vi "SwitchOption.vi"(6 "SubPanelRef":refnum<vi>, 7 "Panel Controller":refnum<class "MemberPanel.lvclass">, 8 "error in (no error)":errorcluster, 9 "Base Path":path, 10 "ThreadName(\"\")":string, 11 "Admin_Actor in":refnum<class "Admin_Actor.lvclass">) -> (0 "error out":errorcluster, 3 "Admin_Actor out":refnum<class "Admin_Actor.lvclass">)   [LabVIEW 2015, in "Admin_Actor.lvlib" / "Admin_Actor.lvclass"]
uses:
  Admin_Actor.lvclass
  Member_Actor/MemberPanel/MemberPanel.lvclass
  Admin_Actor.lvclass/Admin_Actor.ctl
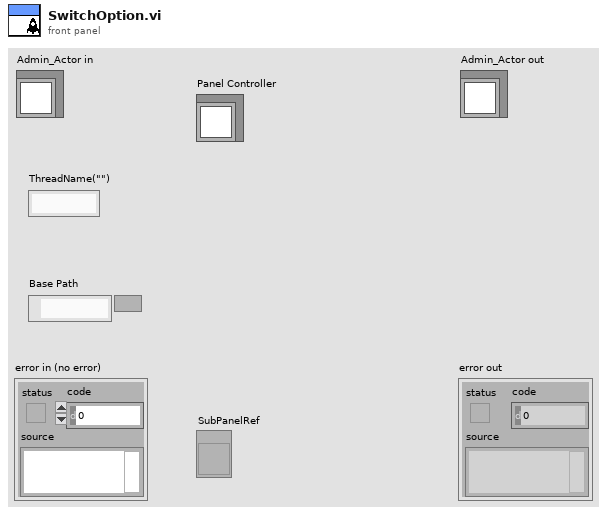
[diagram p1: front panel]
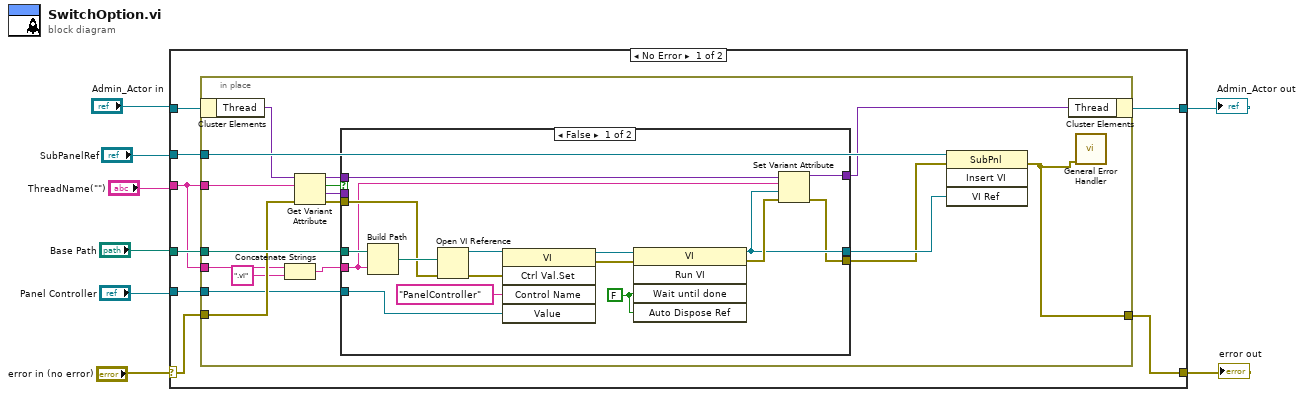
[diagram p0: block diagram]
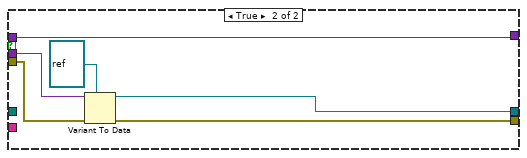
[diagram p2: hidden frame]
diagram:
  n1 = case shown="No Error" "error in (no error)" {
    selector: "error in (no error)" -> [w11 w57]
    tunnel: [w14 w57] -> w4
    tunnel: [w10 w56] -> w1
    tunnel: "Admin_Actor in" -> [w13 w56]
    tunnel: "Base Path" -> [w16 _]
    tunnel: "ThreadName(\"\")" -> [w12 _]
    tunnel: "SubPanelRef" -> [w15 _]
    tunnel: "Panel Controller" -> [w9 _]
    frame No Error {
      n2 = in-place {
        in-place-border: w16 -> [w33]
        in-place-border: w12 -> [w20]
        in-place-border: w15 -> [w32]
        in-place-border: [w17] -> w14
        in-place-border: w12 -> [w28]
        in-place-border: w11 -> [w27]
        in-place-border: w9 -> [w21]
        n3 = in-place-cluster #1(w13) -> ("Thread"=w29:variant)
        n4 = Concatenate Strings(w20, ".vi" ("string")) -> (w18:string)
        n5 = Get Variant Attribute(Variant=w29, name=w28, error in=w27) -> (duplicate Variant=w24:variant, found=w26:bool, value=w23:variant, error out=w25:errorcluster)  [unwired: 1 in]
        n6 = case shown="False" w26 {
          tunnel: w33 -> [w49 _]
          tunnel: w18 -> [w42 _]
          tunnel: [w43 w52] -> w31
          tunnel: [w41 w51] -> w30
          tunnel: w25 -> [w46 w54]
          tunnel: w24 -> [w45 w50]
          tunnel: [w40 w50] -> w22
          tunnel: w23 -> [_ w55]
          tunnel: w21 -> [w34 _]
          frame False {
            w47 = FALSE ("Wait Until Done")
            n7 = Build Path(base path=w49, name or relative path=w42) -> (appended path=w48:path)
            n8 = Open VI Reference(vi path=w48, error in (no error)=w46) -> (vi reference=w39:refnum<vi>, error out=w38:errorcluster)  [unwired: 4 in]
            n9 = invoke class="VI" method="Ctrl Val.Set"(reference=w39, error in=w38, "Control Name"="PanelController", "Value"=w34) -> (reference out=w36:refnum<vi>, error out=w37:errorcluster)  [unwired: 1 in, 3 out]
            n10 = invoke class="VI" method="Run VI"(reference=w36, error in=w37, "Wait until done"=w47, "Auto Dispose Ref"=w47) -> (reference out=w43:refnum<vi>, error out=w44:errorcluster)  [unwired: 1 in, 3 out]
            n11 = Set Variant Attribute(Variant=w45, name=w42, value=w43, error in=w44) -> (Variant out=w40:variant, error out=w41:errorcluster)  [unwired: 1 out]
          }
          frame True {
            n12 = Variant To Data(error in=w54, type=refnum<vi> refnum ("vi reference"), Variant=w55) -> (data=w52:refnum<vi>, error out=w51:errorcluster)
          }
        }
        n13 = invoke class="SubPnl" method="Insert VI"(reference=w32, error in=w30, "VI Ref"=w31) -> (error out=w17:errorcluster)  [unwired: 1 in, 3 out]
        n14 = in-place-cluster #1("Thread"=w22) -> (w10:refnum<class "Admin_Actor.lvclass">)
        n15 = call <vilib>:"General Error Handler.vi"("error in (no error)"=w17) -> ()  [unwired: 10 in, 5 out]
      }
    }
    frame Error {
    }
  }
  "error out" <- w4
  "Admin_Actor out" <- w1
